vi "Enum mode to string for Documentation.vi"() -> ()   [LabVIEW 2009]
panel:
  out "trimmed string":string
  in  "Mode":T1(ring)=enum."Start Grab"
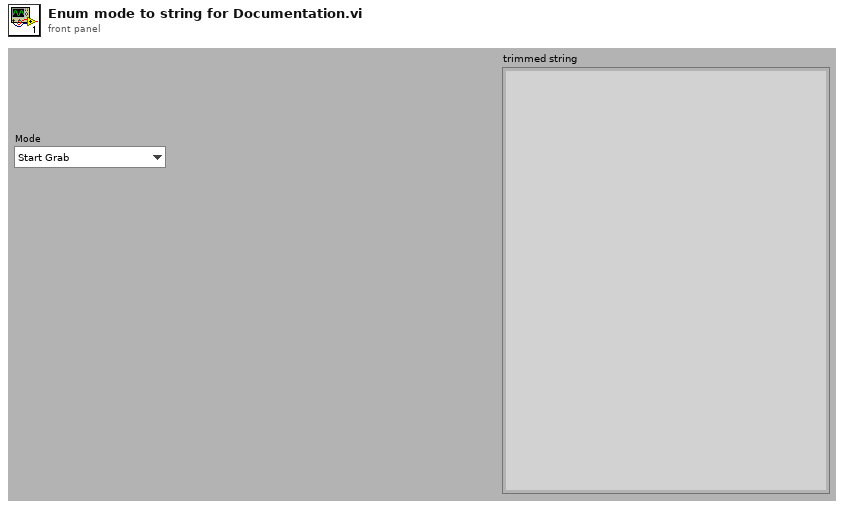
[diagram p1: front panel]
types:
  T1 = enum16{"Open", "Camera Info", "Configure Camera", "Set Cam mode", "Set Shutter", "Set Height", "Set ROI", "Set Width", "Set Rate", "Set Offset and Gain", "Set Trigger Mode", "Read Trigger Line", "Start Grab", "Grab", "Stop Grab", "Start Ring Acq", "Get Ring Buf", "Stop Ring Acq", "Send Serial CMD", "Close"}
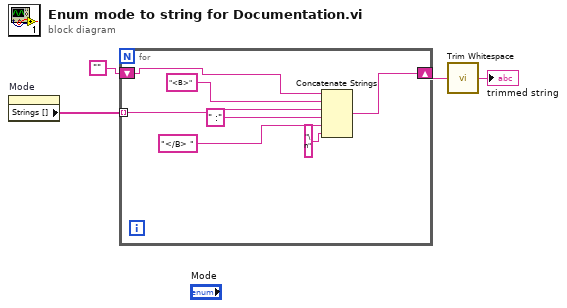
[diagram p0: block diagram]
diagram:
  n1 = property on="Mode" class="Enum (strict)"() -> ("Strings []"=w4:string[])  [unwired: 2 in, 2 out]
  n2 = for {
    tunnel: w4 -> [w11] mode=indexing
    shift-right: [w5] -> w2
    shift-left: "" -> [w6]
    n3 = Concatenate Strings(w6, "<B>" ("string"), w11, " :" ("string"), "</B> " ("string"), "\n" ("string")) -> (w5:string)
  }
  n4 = call <vilib>:"Trim Whitespace.vi"("string"=w2) -> ("trimmed string"=→"trimmed string":string)  [unwired: 1 in]
